vi "Get Buffer.vi"(8 "error in (no error)":errorcluster, 11 "CConfig Buffer Type":refnum<class "CConfig Buffer Type.lvclass">) -> (0 "error out":errorcluster, 1 "Copy data?":bool, 2 "Config":refnum<class "Carya Config.lvclass">, 3 "CConfig Buffer Type":refnum<class "CConfig Buffer Type.lvclass">)   [LabVIEW 2013, in "CConfig Buffer Type.lvclass"]
doc: "Copyright 2018, Carya Automatisering, Wiebe Walstra."
uses:
  CConfig Buffer Type.lvclass
  Carya Config.lvclass
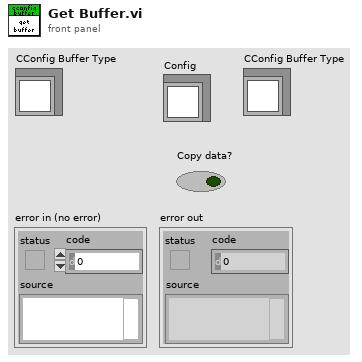
[diagram p1: front panel]
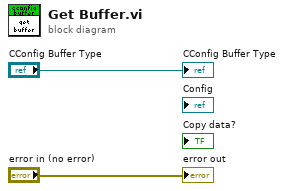
[diagram p0: block diagram]
diagram:
  "error out" <- "error in (no error)"
  "CConfig Buffer Type" <- "CConfig Buffer Type"
